vi "Main.vi"() -> ()   [LabVIEW 2021]
doc: "The myRIO Project template acquires acceleration data from the onboard accelerometer and displays the changes of acceleration values in a waveform chart."
uses:
  <vilib>/userDefined/High Color/IMAQdx.ctl
  <vilib>/vision/Shape Detection.llb/ShapeDetectionMatchOptions.ctl
  <vilib>/vision/Pattern Matching.llb/IMAQ Match Range Setting.ctl
  <vilib>/vision/driver/IMAQdx.llb/IMAQdx Acquisition Mode.ctl
  <vilib>/vision/driver/IMAQdx.llb/IMAQdx Buffer Number Mode.ctl
  <vilib>/vision/Management.llb/Cast Image 2 Method.ctl
  <vilib>/myRIO/Common/Instrument Driver Framework/myRIO v1.0/UART/vis/myRIO v1.0 Close UART.vi
  <vilib>/myRIO/Common/Instrument Driver Framework/Utilities/vis/FPGA Ref Manager.vi
  <vilib>/myRIO/Common/Instrument Driver Framework/myRIO v1.0/myRIO v1.0 Reset FPGA.vi
  <vilib>/myRIO/Common/Instrument Driver Framework/myRIO v1.0/IRQ/vis/myRIO v1.0 IRQ Info FGV.vi
  <vilib>/myRIO/Common/Instrument Driver Framework/myRIO v1.0/IRQ/vis/myRIO v1.0 Timer IRQ Info FGV.vi
  <vilib>/myRIO/Common/Instrument Driver Framework/myRIO v1.0/IRQ/vis/myRIO v1.0 ISR Agent.vi
  <vilib>/myRIO/Instrument Drivers/Utilities/vis/Reset Index.vi
  <vilib>/myRIO/Common/Instrument Driver Framework/myRIO v1.0/Resource Manager/vis/myRIO v1.0 Block Write Resource Manager.vi
  <vilib>/vision/driver/NI_Vision_Acquisition_Software.lvlib
  <vilib>/vision/NI_Vision_Development_Module.lvlib
  <vilib>/myRIO/Instrument Drivers/Utilities/Utilities.lvlib
panel:
  out "XY Graph":cluster{"X":sgl, "Y":sgl}[](graph)
  out "array":cluster{"X":sgl, "Y":sgl}[](array[cluster])
  out "error out":errorcluster
  in  "Circle Descriptor":cluster{"Min Radius":dbl, "Max Radius":dbl}={"Min Radius"=3.0, "Max Radius"=500.0}
  in  "Match Options":T1 {"Range Settings"."Match Constraints" items=["Rotation Angle (degrees)", "Scale Factor (%)", "Occlusion (%)"]}
  in  "Rectangle":T3 {"Rotation" min=-90.0 max=90.0 step=1.0 format="%.2f"; "Left" scale=0.0..1024.0; "Right" scale=0.0..1024.0}
  in  "Session In":T4
  # "Overview: The myRIO Project template acquires acceleration data from the onboard accelerometer and displays the changes of acceleration values in a waveform chart.\nInstructions:\n1. Check the myRIO target IP address in the project and make sure the target IP address is correct. \n2. Run this VI."
  # "Range"
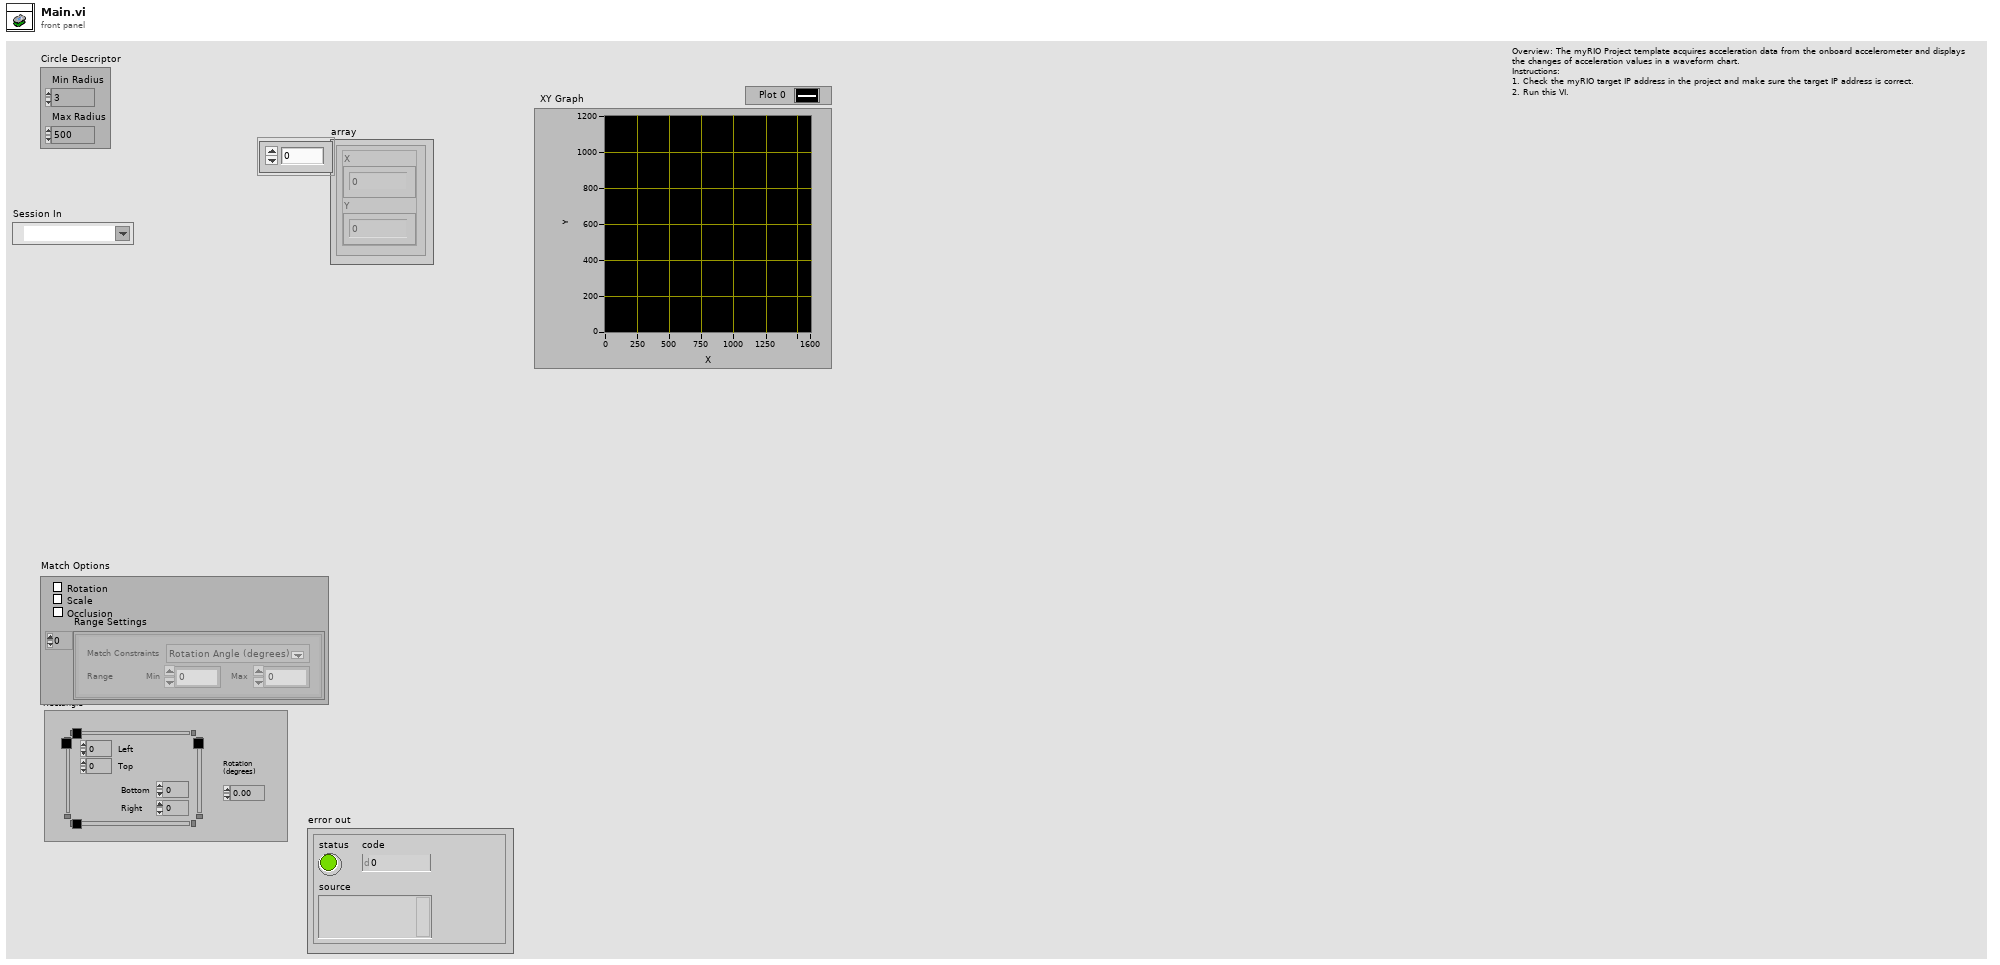
[diagram p1: front panel]
types:
  T1 = typedef "ShapeDetectionMatchOptions.ctl" = cluster{"Rotation":bool, "Scale":bool, "Occlusion":bool, "Range Settings":T2[]}
  T2 = typedef "IMAQ Match Range Setting.ctl" = cluster{"Match Constraints":u32, "Min":dbl, "Max":dbl}
  T3 = typedef "IMAQ Rectangle" = cluster{"Left":i32, "Top":i32, "Right":i32, "Bottom":i32, "Rotation":dbl}
  T4 = typedef "IMAQdx.ctl" = refnum<k21>
  T5 = typedef "NI_Vision_Acquisition_Software.lvlib/IMAQdx Acquisition Mode.ctl" = enum32{"One Shot", "Continuous"}
  T6 = typedef "NI_Vision_Acquisition_Software.lvlib/IMAQdx Buffer Number Mode.ctl" = enum32{"Next", "Last", "Buffer Number", "Every", "Last New"}
  T7 = typedef "Image Type" = u32
  T8 = typedef "IMAQ Image.ctl" = refnum<image>
  T9 = typedef "Cast Image 2 Method.ctl" = u32
  T10 = typedef "ROI Descriptor" = cluster{"Global Rectangle":i32[], "Contours":cluster{"ID":enum32{"External", "Internal"}, "Type":u32, "Coordinates":i32[]}[]}
  T11 = cluster{"Position":cluster{"X":sgl, "Y":sgl}, "Radius":dbl, "Score":dbl}[]
  T12 = cluster{"Circles[0]":cluster{"Position":cluster{"X":sgl, "Y":sgl}, "Radius":dbl, "Score":dbl}, "Circles[1]":cluster{"Position":cluster{"X":sgl, "Y":sgl}, "Radius":dbl, "Score":dbl}, "Circles[2]":cluster{"Position":cluster{"X":sgl, "Y":sgl}, "Radius":dbl, "Score":dbl}, "Circles[3]":cluster{"Position":cluster{"X":sgl, "Y":sgl}, "Radius":dbl, "Score":dbl}, "Circles[4]":cluster{"Position":cluster{"X":sgl, "Y":sgl}, "Radius":dbl, "Score":dbl}, "Circles[5]":cluster{"Position":cluster{"X":sgl, "Y":sgl}, "Radius":dbl, "Score":dbl}, "Circles[6]":cluster{"Position":cluster{"X":sgl, "Y":sgl}, "Radius":dbl, "Score":dbl}, "Circles[7]":cluster{"Position":cluster{"X":sgl, "Y":sgl}, "Radius":dbl, "Score":dbl}, "Circles[8]":cluster{"Position":cluster{"X":sgl, "Y":sgl}, "Radius":dbl, "Score":dbl}}
  T13 = cluster{"Position":cluster{"X":sgl, "Y":sgl}, "Radius":dbl, "Score":dbl}
  T14 = cluster{"Position":cluster{"X":sgl, "Y":sgl}, "Position":cluster{"X":sgl, "Y":sgl}, "Position":cluster{"X":sgl, "Y":sgl}, "Position":cluster{"X":sgl, "Y":sgl}, "Position":cluster{"X":sgl, "Y":sgl}, "Position":cluster{"X":sgl, "Y":sgl}, "Position":cluster{"X":sgl, "Y":sgl}, "Position":cluster{"X":sgl, "Y":sgl}, "Position":cluster{"X":sgl, "Y":sgl}}
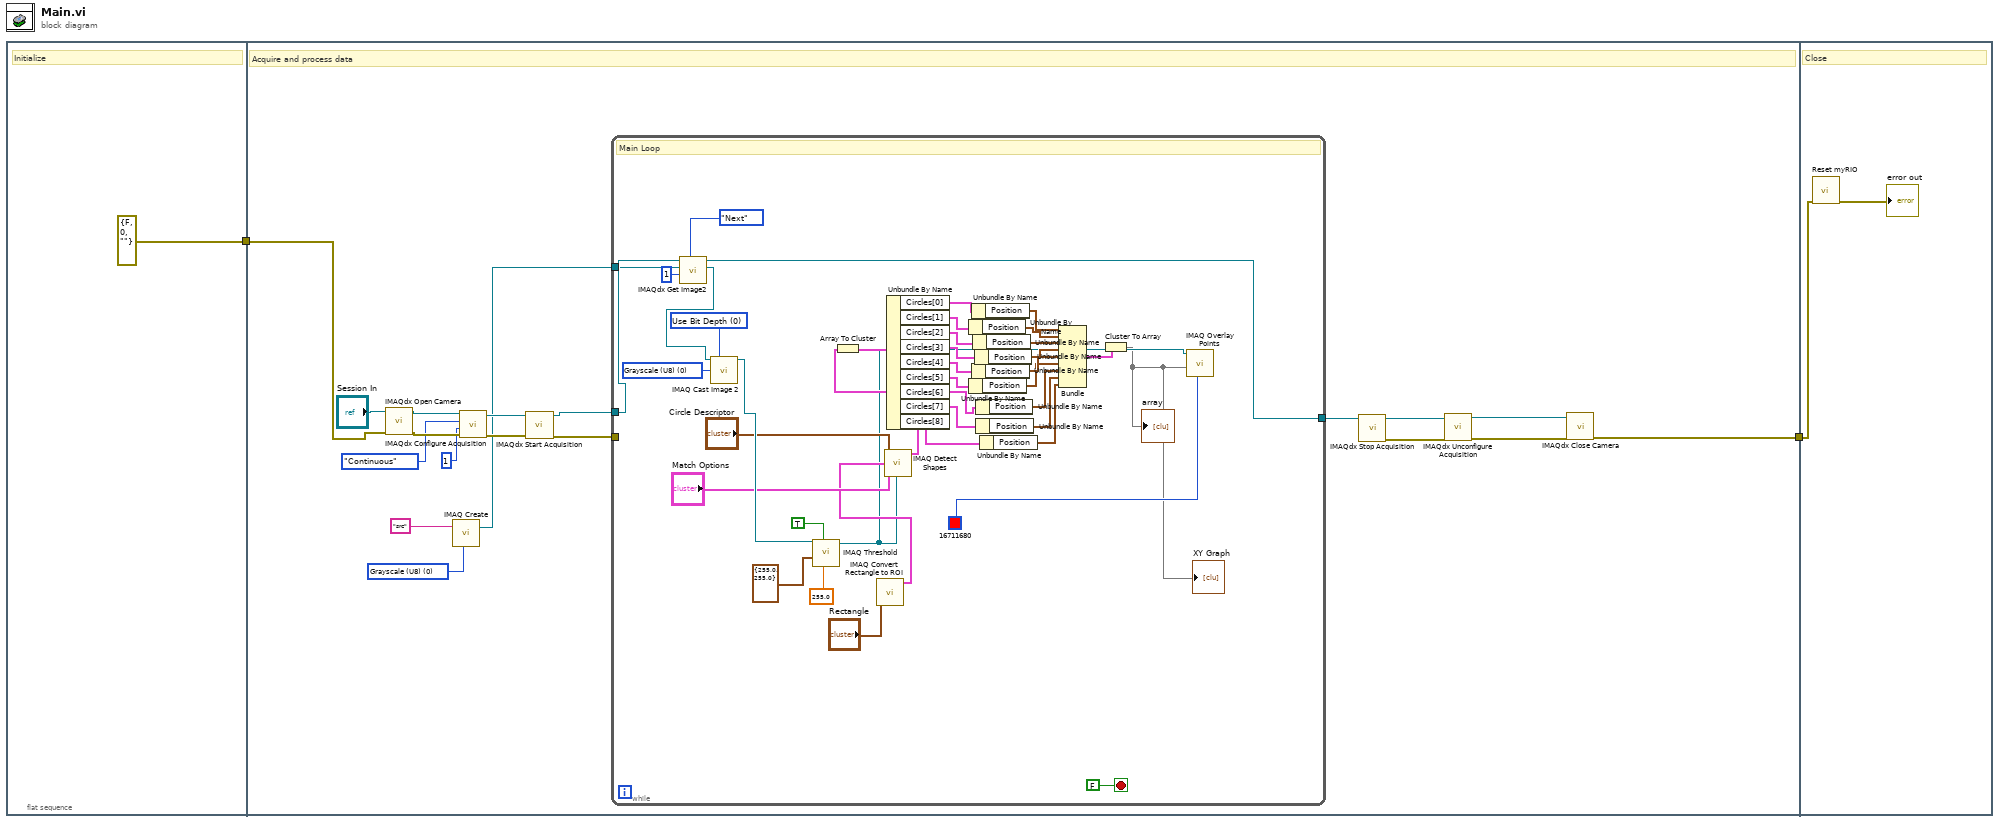
[diagram p0: block diagram]
diagram:
  n1 = flat-sequence {
    tunnel: [errorcluster {"status"=FALSE, "code"=0, "source"=""} ("error in")] -> w2
    tunnel: [w9] -> w1
    tunnel: w2 -> [w8]
    tunnel: w1 -> [w64]
    frame #0 {
      # "Initialize"
    }
    frame #1 {
      w5 = T7 0 items=["Grayscale (U8)", "Grayscale (I16)", "Grayscale (SGL)", "Complex (CSG)", "RGB (U32)", "HSL (U32)", "RGB (U64)", "Grayscale (U16)"] ("Image Type")
      # "Acquire and process data"
      n2 = call <vilib>:"IMAQdx Open Camera.vi"("error in"=w8, "Session In"="Session In") -> ("error out"=w13:errorcluster, "Session Out"=w14:T4)  [unwired: 8 in]
      n3 = call "IMAQ Create"("Image Name"="src", "Image Type"=w5) -> ("New Image"=w4:T8)  [unwired: 3 in, 1 out]
      n4 = call <vilib>:"IMAQdx Configure Acquisition.vi"("error in"=w13, "Number of Buffers"=u32 1, "Continuous?"=IMAQdx_Acquisition_Mode."Continuous", "Session In"=w14) -> ("error out"=w22:errorcluster, "Session Out"=w21:T4)  [unwired: 6 in]
      n5 = call <vilib>:"IMAQdx Start Acquisition.vi"("error in"=w22, "Session In"=w21) -> ("error out"=w20:errorcluster, "Session Out"=w19:T4)  [unwired: 8 in]
      n6 = while {
        tunnel: w19 -> [w26]
        tunnel: w20 -> [_]
        tunnel: [w28] -> w7
        tunnel: w4 -> [w25]
        stop <- FALSE stop-if-true
        w59 = T9 0 items=["Use Bit Depth", "Shift", "Use Lookup Table"] ("Method")
        w60 = T7 0 items=["Grayscale (U8)", "Grayscale (I16)", "Grayscale (SGL)", "Complex (CSG)", "RGB (U32)", "HSL (U32)", "RGB (U64)", "Grayscale (U16)"] ("Image Type")
        # "Main Loop"
        n7 = call <vilib>:"IMAQdx Get Image2.vi"("Buffer Number Mode (Next)"=IMAQdx_Buffer_Number_Mode."Next", "Buffer Number In"=u32 1, "Image In"=w25, "Session In"=w26) -> ("Image Out"=w58:T8, "Session Out"=w28:T4)  [unwired: 4 in, 2 out]
        n8 = call "IMAQ Cast Image 2"("Image Src"=w58, "Method"=w59, "Image Type"=w60) -> ("Image Dst Out"=w57:T8)  [unwired: 11 in, 1 out]
        n9 = call "IMAQ Threshold"("Replace Value"=sgl 255.0, "Keep/Replace Value (Replace)"=TRUE, "Range"=cluster{"Upper value":sgl, "Lower value":sgl} {"Upper value"=255.0, "Lower value"=255.0}, "Image Src"=w57) -> ("Image Dst Out"=w35:T8)  [unwired: 6 in, 1 out]
        n10 = call "IMAQ Convert Rectangle to ROI"("Rectangle"="Rectangle") -> ("ROI Descriptor"=w48:T10)  [unwired: 8 in, 1 out]
        n11 = call-poly "IMAQ Detect Shapes"("ROI Descriptor"=w48, "Match Options"="Match Options", "Circle Descriptor"="Circle Descriptor", "Image"=w35) -> ("Circles"=w52:T11)  [unwired: 5 in, 2 out]
        n12 = Array To Cluster(array=w52) -> (cluster=w51:T12)
        n13 = Unbundle By Name(w51) -> ("Circles[0]"=w50:T13, "Circles[1]"=w47:T13, "Circles[2]"=w46:T13, "Circles[3]"=w45:T13, "Circles[4]"=w44:T13, "Circles[5]"=w43:T13, "Circles[6]"=w34:T13, "Circles[7]"=w33:T13, "Circles[8]"=w32:T13)
        n14 = Unbundle By Name(w47) -> ("Position"=w41:cluster{"X":sgl, "Y":sgl})
        n15 = Unbundle By Name(w43) -> ("Position"=w37:cluster{"X":sgl, "Y":sgl})
        n16 = Unbundle By Name(w50) -> ("Position"=w42:cluster{"X":sgl, "Y":sgl})
        n17 = Unbundle By Name(w44) -> ("Position"=w38:cluster{"X":sgl, "Y":sgl})
        n18 = Unbundle By Name(w46) -> ("Position"=w40:cluster{"X":sgl, "Y":sgl})
        n19 = Unbundle By Name(w45) -> ("Position"=w39:cluster{"X":sgl, "Y":sgl})
        n20 = Unbundle By Name(w34) -> ("Position"=w31:cluster{"X":sgl, "Y":sgl})
        n21 = Unbundle By Name(w33) -> ("Position"=w30:cluster{"X":sgl, "Y":sgl})
        n22 = Unbundle By Name(w32) -> ("Position"=w29:cluster{"X":sgl, "Y":sgl})
        n23 = Bundle("Position"=w42, "Position"=w41, "Position"=w40, "Position"=w39, "Position"=w38, "Position"=w37, "Position"=w31, "Position"=w30, "Position"=w29) -> (w36:T14)  [unwired: 1 in]
        n24 = Cluster To Array(cluster=w36) -> (array=w23:cluster{"X":sgl, "Y":sgl}[])
        "array" <- w23
        "XY Graph" <- w23
        n25 = call "IMAQ Overlay Points"("Color"=u32 16711680, "Array of Points"=w23, "Image"=w35) -> ()  [unwired: 7 in, 2 out]
      }
      n26 = call <vilib>:"IMAQdx Stop Acquisition.vi"("Session In"=w7) -> ("error out"=w16:errorcluster, "Session Out"=w15:T4)  [unwired: 9 in]
      n27 = call <vilib>:"IMAQdx Unconfigure Acquisition.vi"("error in"=w16, "Session In"=w15) -> ("error out"=w18:errorcluster, "Session Out"=w17:T4)  [unwired: 8 in]
      n28 = call <vilib>:"IMAQdx Close Camera.vi"("error in"=w18, "Session In"=w17) -> ("error out"=w9:errorcluster)  [unwired: 9 in]
    }
    frame #2 {
      # "Close"
      n29 = call <vilib>:"Reset myRIO.vi"("error in (no error)"=w64) -> ("error out"=→"error out":errorcluster)  [unwired: 10 in]
    }
  }
